vi "Do.vi"(6 "CMD":T1, 8 "error in (no error)":errorcluster, 10 "Do":bool, 11 "Valve_2DO_2DI in":refnum<class "Valve_2DO_2DI.lvclass">) -> (0 "error out":errorcluster, 2 "Done":bool, 3 "Valve_2DO_2DI out":refnum<class "Valve_2DO_2DI.lvclass">)   [LabVIEW 2019, in "Valve_2DO_2DI.lvclass"]
uses:
  Valve_2DO_2DI.lvclass
  CMD.ctl
  Valve_2DO_2DI.lvclass/Valve_2DO_2DI.ctl
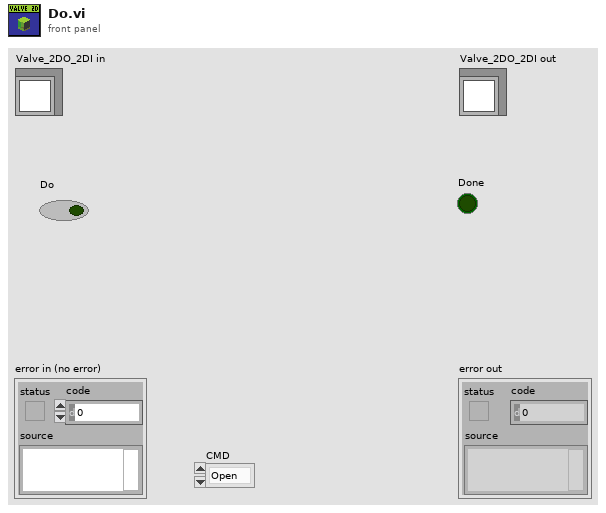
[diagram p1: front panel]
types:
  T1 = typedef "Valve_2DO_2DI.lvclass/CMD.ctl" = enum16{"Open", "Close"}
  T2 = typedef "valveState.ctl" = enum16{"Unknown", "Closed", "Opening", "Opened", "Closing"}
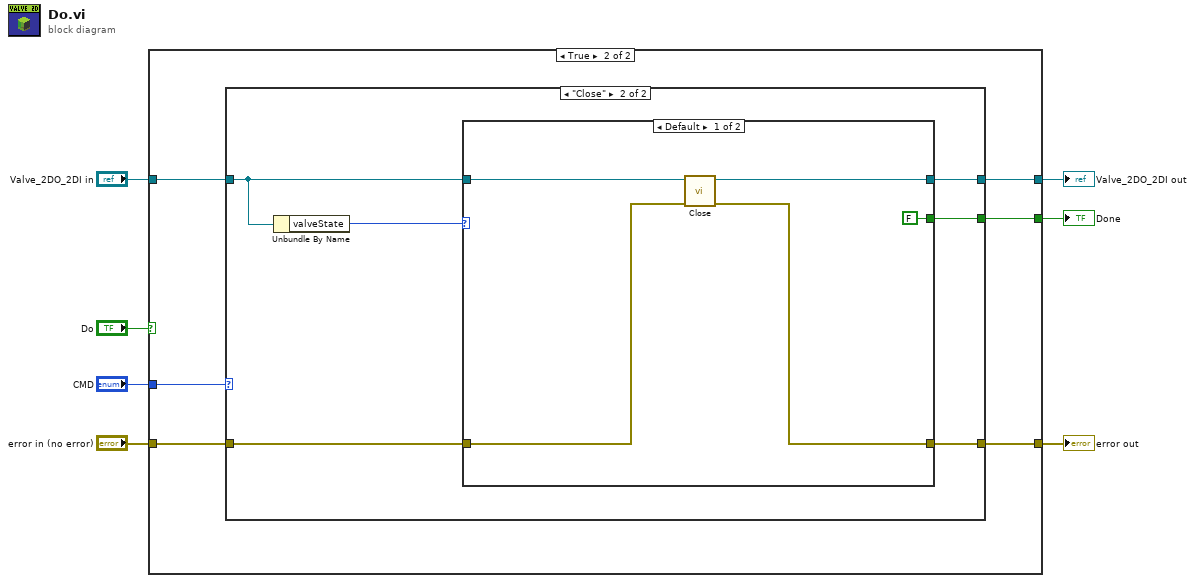
[diagram p0: block diagram]
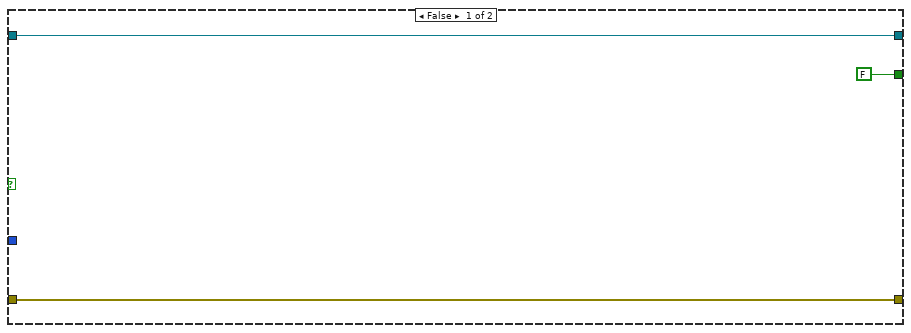
[diagram p2: hidden frame]
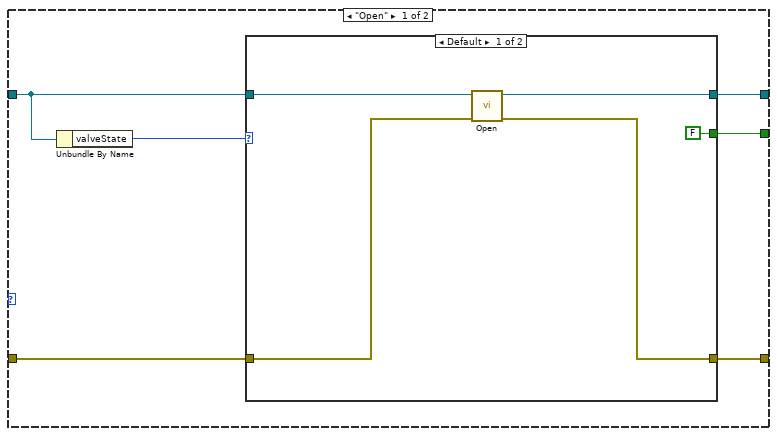
[diagram p3: hidden frame]
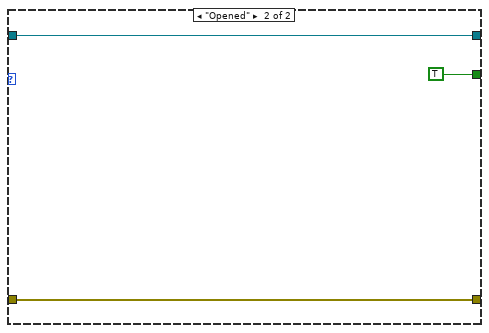
[diagram p4: hidden frame]
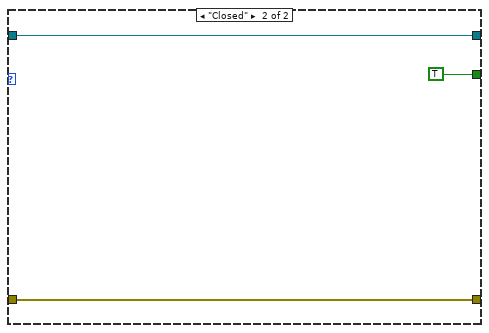
[diagram p5: hidden frame]
diagram:
  n1 = case shown="True" "Do" {
    tunnel: [w10 w14] -> w7
    tunnel: "Valve_2DO_2DI in" -> [w10 w15]
    tunnel: [w8 w12] -> w4
    tunnel: "error in (no error)" -> [w8 w11]
    tunnel: [FALSE ("Done") w13] -> w2
    tunnel: "CMD" -> [_ w16]
    frame False {
    }
    frame True {
      n2 = case shown="\"Close\"" w16 {
        tunnel: w15 -> [w20 w34]
        tunnel: [w21 w35] -> w14
        tunnel: [w19 w33] -> w13
        tunnel: [w18 w32] -> w12
        tunnel: w11 -> [w17 w31]
        frame "Open" {
          n3 = Unbundle By Name(w20) -> ("valveState"=w22:T2)
          n4 = case shown="Default" w22 {
            tunnel: [w25 w30] -> w21
            tunnel: w20 -> [w26 w30]
            tunnel: [FALSE TRUE] -> w19
            tunnel: [w23 w28] -> w18
            tunnel: w17 -> [w24 w28]
            frame Default {
              n5 = call "Open.vi"("error in (no error)"=w24, "Pump_1AI_1DO_2DI in"=w26) -> ("error out"=w23:errorcluster, "Pump_1AI_1DO_2DI out"=w25:refnum<class "Valve_2DO_2DI.lvclass">)  [unwired: 8 in]
            }
            frame "Opened" {
            }
          }
        }
        frame "Close" {
          n6 = Unbundle By Name(w34) -> ("valveState"=w36:T2)
          n7 = case shown="Default" w36 {
            tunnel: [w39 w44] -> w35
            tunnel: w34 -> [w40 w44]
            tunnel: [FALSE TRUE] -> w33
            tunnel: [w37 w42] -> w32
            tunnel: w31 -> [w38 w42]
            frame Default {
              n8 = call "Close.vi"("error in (no error)"=w38, "Pump_1AI_1DO_2DI in"=w40) -> ("error out"=w37:errorcluster, "Pump_1AI_1DO_2DI out"=w39:refnum<class "Valve_2DO_2DI.lvclass">)  [unwired: 8 in]
            }
            frame "Closed" {
            }
          }
        }
      }
    }
  }
  "error out" <- w4
  "Valve_2DO_2DI out" <- w7
  "Done" <- w2
